vi "FlatToRichRequest.vi"(5 "OutputClusterType":T1, 11 "InputCluster":T2) -> (3 "OutputCluster":T1)   [LabVIEW 2019, in "Generated_server.lvlib"]
uses:
  Generated_server.lvlib
  Request_Flat.ctl
  Request.ctl
  Request_request_oneof/Request_request_oneof.lvclass
  Request_request_oneof/Request_request_oneof.lvclass/Request_request_oneof.ctl
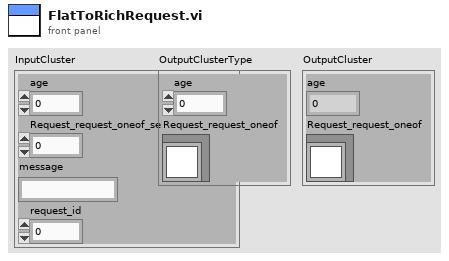
[diagram p1: front panel]
types:
  T1 = typedef "Generated_server.lvlib/Request.ctl" = cluster{"age":i32, "Request_request_oneof":refnum<class "Request_request_oneof.lvclass">}
  T2 = typedef "Generated_server.lvlib/Request_Flat.ctl" = cluster{"age":i32, "Request_request_oneof_selected_index":i32, "message":string, "request_id":i32}
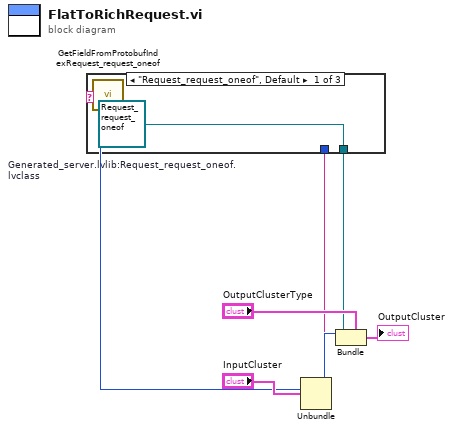
[diagram p0: block diagram]
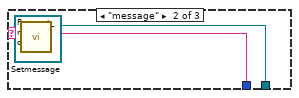
[diagram p2: hidden frame]
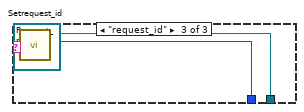
[diagram p3: hidden frame]
diagram:
  n1 = Unbundle "Unbundle"("InputCluster") -> ("age"=w6:i32, "Request_request_oneof_selected_index"=w5:i32, "message"=w2:string, "request_id"=w1:i32)
  n2 = call "GetFieldFromProtobufIndexRequest_request_oneof.vi"("protobuf index"=w5) -> ("oneof field name"=w4:string)
  n3 = case "Request_request_oneof" shown="\"Request_request_oneof\", Default" w4 {
    tunnel: [w10 w12 w15] -> w3
    tunnel: w2 -> [_ w13 _]
    tunnel: w1 -> [_ _ w16]
    frame "Request_request_oneof", Default {
      w10 = refnum<class "Request_request_oneof.lvclass"> refnum  # Generated_server.lvlib:Request_request_oneof.lvclass
    }
    frame "message" {
      n4 = call "Setmessage.vi"("Set_Val"=w13, "OneOfTemplate in"=refnum<class "Request_request_oneof.lvclass"> refnum) -> ("OneOfTemplate out"=w12:refnum<class "Request_request_oneof.lvclass">)  [unwired: 8 in, 1 out]
    }
    frame "request_id" {
      n5 = call "Setrequest_id.vi"("Set_Val"=w16, "OneOfTemplate in"=refnum<class "Request_request_oneof.lvclass"> refnum) -> ("OneOfTemplate out"=w15:refnum<class "Request_request_oneof.lvclass">)  [unwired: 8 in, 1 out]
    }
  }
  n6 = Bundle "Bundle"(cluster="OutputClusterType", "age"=w6, "Request_request_oneof"=w3) -> (→"OutputCluster":T1)
